vi "List JKISM++.vi"(8 "Error in":errorcluster caption="Error in (no error)") -> (0 "Error out":errorcluster, 2 "Name":string[](array[string]), 3 "Array":T1[](array[typedef]))   [LabVIEW 2014, in "JKI-State-Machine-Plus.lvlib"]
uses:
  JKI-State-Machine-Plus.lvlib
  _Support/_JKISMQ.ctl
  _Support/_Cross JKI StateMachine State Data.ctl
  _Support/_Cross JKI StateMachine State Response.ctl
  _Support/_JKISMQFGVOPER.ctl
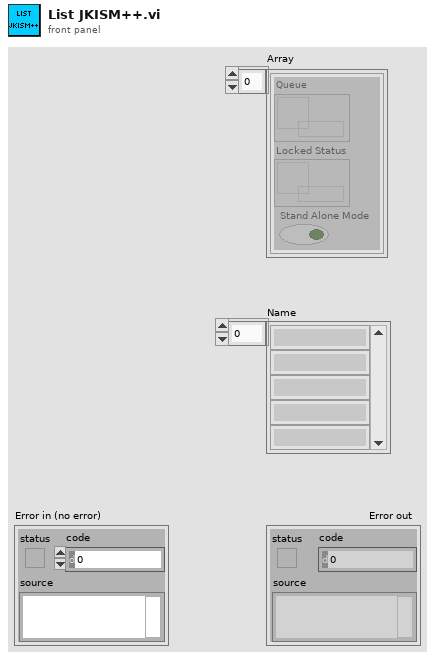
[diagram p1: front panel]
types:
  T1 = typedef "JKI-State-Machine-Plus.lvlib/_JKISMQ.ctl" = cluster{"Queue":refnum<queue>, "Locked Status":refnum<data-value>, "Stand Alone Mode":bool}
  T2 = typedef "JKI-State-Machine-Plus.lvlib/_JKISMQFGVOPER.ctl" = enum16{"Get By Name", "List"}
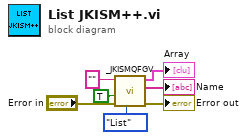
[diagram p0: block diagram]
diagram:
  n1 = call "_JKISMQFGV.vi"("Enum"=_JKISMQFGVOPER."List", "Error in"="Error in", "create if not found? (T)"=TRUE, "Name(\"\" to use uuid) in"="" ("Name(\"\" to use uuid) in")) -> ("Error out"=→"Error out":errorcluster, "Name"=→"Name":string[], "Array"=→"Array":T1[])  [unwired: 5 in]
